vi "rs3_MemCopyUINT16_3.vi"(4 "Depth unit, um/step":i32=1000, 6 "Image format":u16(ring) items=["Y16", "Y8"], 7 "Transpose":bool=TRUE, 8 "error in (no error)":errorcluster, 9 "Depth Y":i32, 10 "Depth X":i32, 11 "Zimage pointer":u64) -> (0 "error out":errorcluster, 1 "Length":i32=10, 2 "2D Array Output":sgl[][](array[numeric]), 3 "Output Array":u16[](array[numeric]))   [LabVIEW 2018, in "libRealSense3.lvlib"]
doc: "Use this after a Get Frame Data VI to copy the memory pointed to, into an 2D array in LabVIEW.\nThis VI should be used for DEPTH and UNRECT IMAGE data that is 16 or 8 bits."
uses:
  libRealSense3.lvlib
panel:
  # "RS3_Mem Copy"
  # "(C) 2017 Intel Corp.,  AGJ"
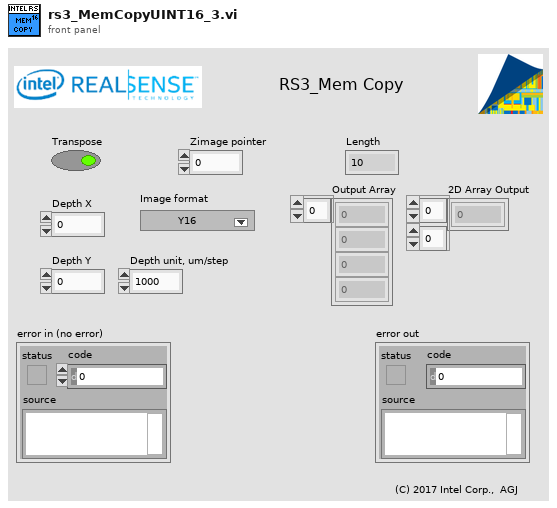
[diagram p1: front panel]
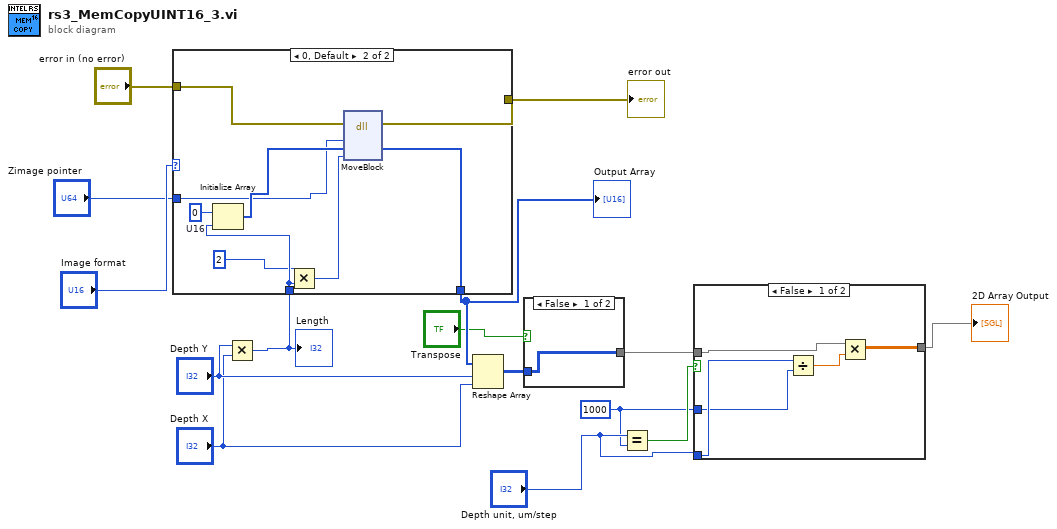
[diagram p0: block diagram]
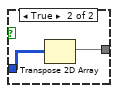
[diagram p2: hidden frame]
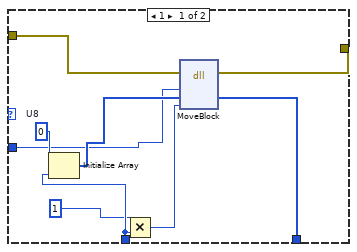
[diagram p4: hidden frame]
diagram:
  w2 = 1000 ("y")
  n1 = Multiply(x="Depth Y", y="Depth X") -> (x*y=w9:i32)
  "Length" <- w9
  n2 = case shown="0, Default" "Image format" {
    tunnel: [w24 w33] -> w14
    tunnel: [w23 w32] -> w13
    tunnel: "error in (no error)" -> [w22 w31]
    tunnel: w9 -> [w18 w27]
    tunnel: "Zimage pointer" -> [w16 w25]
    frame 1 {
      w21 = u8 0  # U8
      n3 = Initialize Array(w21, w18) -> (w20:u8[])
      n4 = Multiply(x=1 ("factor"), y=w18) -> (x*y=w19:i32)
      n5 = dll-call lib="LabVIEW" fn="MoveBlock"(error in=w22, "Address(Pointer)"=w16, "Destination"=w20, "Size"=w19) -> (error out=w23:errorcluster, "Destination"=w24:u8[])  [unwired: 5 in, 1 out]
    }
    frame 0, Default {
      w30 = u16 0  # U16
      n6 = Initialize Array(w30, w27) -> (w29:u16[])
      n7 = Multiply(x=2 ("factor"), y=w27) -> (x*y=w28:i32)
      n8 = dll-call lib="LabVIEW" fn="MoveBlock"(error in=w31, "Address(Pointer)"=w25, "Destination"=w29, "Size"=w28) -> (error out=w32:errorcluster, "Destination"=w33:u16[])  [unwired: 5 in, 1 out]
    }
  }
  "Output Array" <- w14
  "error out" <- w13
  n9 = Reshape Array(w14, "Depth Y", "Depth X") -> (w15:u16[][])
  n10 = case shown="False" "Transpose" {
    tunnel: w15 -> [w34 w36]
    tunnel: [w34 w35] -> w5
    frame False {
    }
    frame True {
      n11 = Transpose 2D Array(2D array=w36) -> (transposed array=w35:u16[][])
    }
  }
  n12 = Equal?(x="Depth unit, um/step", y=w2) -> (x = y?=w6:bool)
  n13 = case shown="False" w6 {
    tunnel: [w38 w42] -> w4
    tunnel: w5 -> [w39 w42]
    tunnel: "Depth unit, um/step" -> [w41 _]
    tunnel: w2 -> [w40 _]
    frame False {
      n14 = Divide(x=w41, y=w40) -> (x/y=w37:dbl)
      n15 = Multiply(x=w39, y=w37) -> (x*y=w38:dbl[][])
    }
    frame True {
    }
  }
  "2D Array Output" <- w4
